vi "FRIC_navX_Get_Displacement.vi"(5 "Device Number":T1, 7 "Update":bool) -> (2 "Displacement":T2)   [LabVIEW 2016]
doc: "This navX VI returns the velocity and displacement of the navX. This VI is only supported on firmware virsions newer than 2.2.xxx."
uses:
  _TypeDefs/FRIC_navX_DeviceNumbersTypeDef.ctl
  _TypeDefs/FRIC_navX_DecodeRegisterLengthClusterTypeDef_.ctl
  _TypeDefs/Z900_navX_DeviceRegisters.ctl
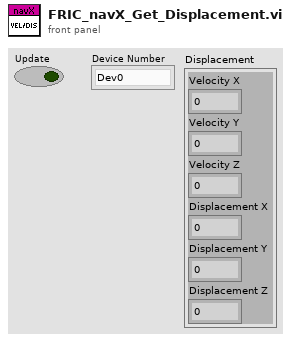
[diagram p1: front panel]
types:
  T1 = typedef "FRIC_navX_DeviceNumbersTypeDef.ctl" = enum16{"Dev0", "Dev1", "Dev2", "Dev3", "Dev4", "Dev5", "Dev6", "Dev7", "Dev8", "Dev9", "Dev10"}
  T2 = cluster{"Velocity X":dbl, "Velocity Y":dbl, "Velocity Z":dbl, "Displacement X":dbl, "Displacement Y":dbl, "Displacement Z":dbl}
  T3 = typedef "FRIC_navX_DecodeRegisterLengthClusterTypeDef_.ctl" = cluster{"Device Register":T4, "length":i32}[]
  T4 = typedef "Z900_navX_DeviceRegisters.ctl" = u8
  T5 = cluster{"Velocity X":dbl, "Velocity Y":dbl, "Velocity Z":dbl, "Displacement X":dbl, "Displacement Y":dbl, "Displacement Z":dbl}[]
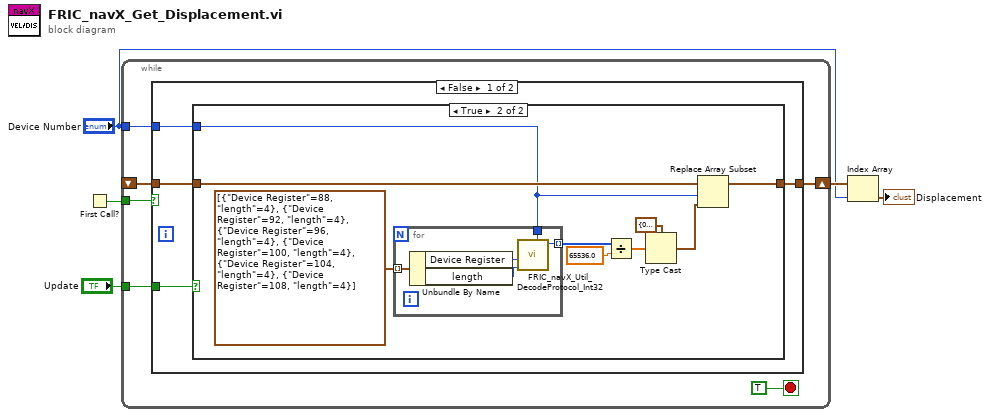
[diagram p0: block diagram]
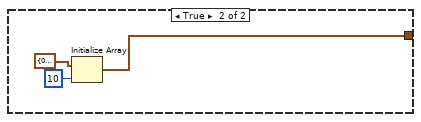
[diagram p3: hidden frame]
diagram:
  n1 = First Call?() -> (First Call?: T/F=w1:bool)
  n2 = while {
    shift-right: [w11] -> w4
    shift-left: _ -> [w9]
    tunnel: "Update" -> [w8]
    tunnel: "Device Number" -> [w7]
    tunnel: w1 -> [w6]
    stop <- TRUE stop-if-true
    n3 = case shown="False" w6 {
      tunnel: [w15 w31] -> w11
      tunnel: w9 -> [w14 _]
      tunnel: w8 -> [w12 _]
      tunnel: w7 -> [w13 _]
      frame False {
        n4 = case shown="True" w12 {
          tunnel: [w16 w18] -> w15
          tunnel: w14 -> [w16 w19]
          tunnel: w13 -> [_ w17]
          frame False {
          }
          frame True {
            n5 = for {
              tunnel: T3 [{"Device Register"=88, "length"=4}, {"Device Register"=92, "length"=4}, {"Device Register"=96, "length"=4}, {"Device Register"=100, "length"=4}, {"Device Register"=104, "length"=4}, {"Device Register"=108, "length"=4}] -> [w30] mode=indexing
              tunnel: [w27] -> w22 mode=indexing
              tunnel: w17 -> [w26]
              n6 = Unbundle By Name(w30) -> ("Device Register"=w29:T4, "length"=w28:i32)
              n7 = call "FRIC_navX_Util_DecodeProtocol_Int32.vi"("Device Number"=w26, "length"=w28, "Device Register"=w29) -> ("Value"=w27:i32)  [unwired: 7 in]
            }
            n8 = Divide(x=w22, y=65536.0) -> (x/y=w21:dbl[])
            n9 = Type Cast(type=T2 {"Velocity X"=0.0, "Velocity Y"=0.0, "Velocity Z"=0.0, "Displacement X"=0.0, "Displacement Y"=0.0, "Displacement Z"=0.0}, x=w21) -> (*(type *) &x=w20:T2)
            n10 = Replace Array Subset(array=w19, new element=w20, index=w17) -> (w18:T5)
          }
        }
      }
      frame True {
        n11 = Initialize Array(T2 {"Velocity X"=0.0, "Velocity Y"=0.0, "Velocity Z"=0.0, "Displacement X"=0.0, "Displacement Y"=0.0, "Displacement Z"=0.0}, 10 ("dimension size")) -> (w31:T5)
      }
    }
  }
  n12 = Index Array(array=w4, index="Device Number") -> (element=→"Displacement":T2)
